vi "NRZ decoder.vi"(8 "error in (no error)":errorcluster, 11 "Bit stream in":u8[](array[numeric])) -> (0 "error out":errorcluster, 3 "Array":u8[](array[numeric]))   [LabVIEW 2019]
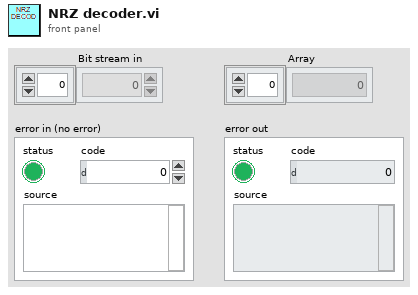
[diagram p1: front panel]
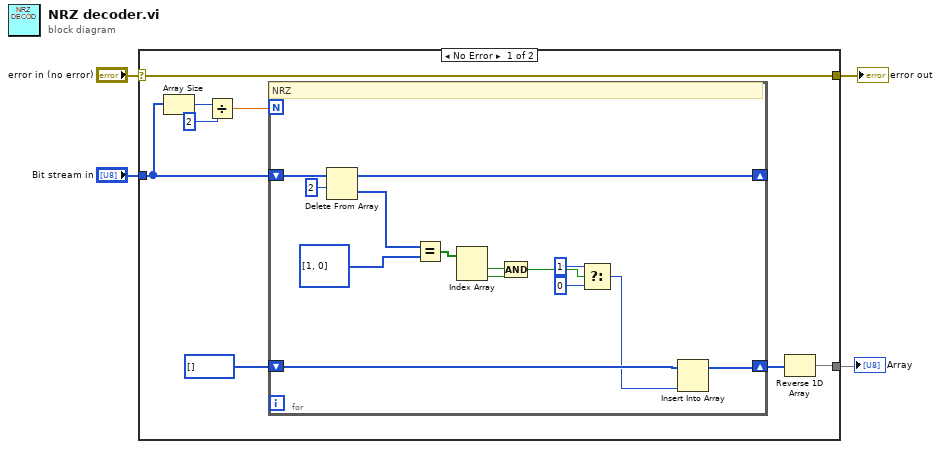
[diagram p0: block diagram]
diagram:
  n1 = case shown="No Error" "error in (no error)" {
    selector: "error in (no error)" -> [w12 w27]
    tunnel: "Bit stream in" -> [w8 _]
    tunnel: [w12 w27] -> w2
    tunnel: [w7 _] -> w1
    frame No Error {
      n2 = Array Size(array=w8) -> (size(s)=w11:i32)
      n3 = Divide(x=w11, y=2) -> (x/y=w5:dbl)
      n4 = for {
        N: w5 -> [_]
        shift-right: [w14] -> w6
        shift-left: u8[] [] ("output array") -> [w15]
        shift-right: [w24] -> _
        shift-left: w8 -> [w26]
        # "NRZ"
        n5 = Delete From Array(array=w26, length=2) -> (deleted portion=w20:u8[], array with subset deleted=w24:u8[])  [unwired: 1 in]
        n6 = Equal?(x=w20, y=u8[] [1, 0] ("output array")) -> (x = y?=w19:bool[])
        n7 = Index Array(array=w19) -> (element #1=w18:bool, element #2=w17:bool)  [unwired: 2 in]
        n8 = Compound Arithmetic op=AND(w18, w17) -> (w16:bool)
        n9 = Select(t=u8 1, s=w16, f=u8 0) -> (s? t:f=w13:u8)
        n10 = Insert Into Array(array=w15, new element=w13) -> (w14:u8[])  [unwired: 1 in]
      }
      n11 = Reverse 1D Array(array=w6) -> (reversed array=w7:u8[])
    }
    frame Error {
    }
  }
  "error out" <- w2
  "Array" <- w1
